vi "Boolean Array to Selected Element.vi"(7 "Bool Array In":bool[](array[boolean])) -> (8 "Selected Element Out":i32)   [LabVIEW 2016, in "TLMB.lvlib"]
uses:
  Projects/TLMB.lvlib
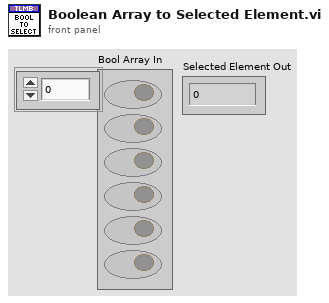
[diagram p1: front panel]
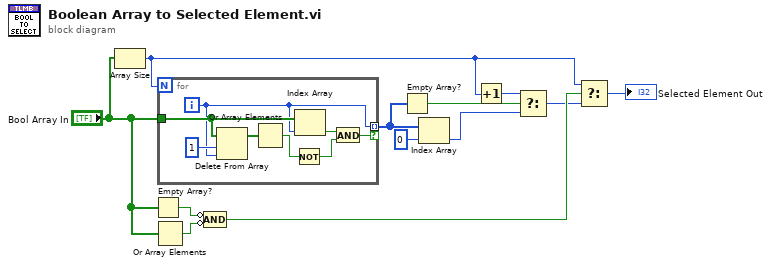
[diagram p0: block diagram]
diagram:
  n1 = Array Size(array="Bool Array In") -> (size(s)=w2:i32)
  n2 = Empty Array?(array="Bool Array In") -> (empty?=w9:bool)
  n3 = Or Array Elements(Boolean array="Bool Array In") -> (logical OR=w8:bool)
  n4 = for {
    N: w2 -> [_]
    tunnel: "Bool Array In" -> [w20]
    tunnel: [w15] -> w11 mode=indexing if=w14
    i -> [w15]
    n5 = Delete From Array(array=w20, length=1, index=w15) -> (array with subset deleted=w13:bool[])  [unwired: 1 out]
    n6 = Or Array Elements(Boolean array=w13) -> (logical OR=w18:bool)
    n7 = Not(x=w18) -> (.not. x?=w17:bool)
    n8 = Index Array(array=w20, index=w15) -> (element=w16:bool)
    n9 = And(x=w16, y=w17) -> (x .and. y?=w14:bool)
  }
  n10 = Compound Arithmetic op=AND(invert w9, invert w8) -> (w7:bool)
  n11 = Empty Array?(array=w11) -> (empty?=w5:bool)
  n12 = Index Array(array=w11, index=0) -> (element=w6:i32)
  n13 = Increment(x=w2) -> (x+1=w1:i32)
  n14 = Select(t=w1, s=w5, f=w6) -> (s? t:f=w4:i32)
  n15 = Select(t=w2, s=w7, f=w4) -> (s? t:f=→"Selected Element Out":i32)
